vi "Connect.vi"(8 "error in (no error)":errorcluster) -> (0 "error out":errorcluster, 2 "controller":refnum<k24>)   [LabVIEW 2016]
uses:
  C:/Program Files (x86)/Aerotech/A3200/LabVIEW/2010/Bin/Aerotech.A3200.dll
  Program Files (x86)/Aerotech/A3200/LabVIEW/2010/Bin/Aerotech.A3200.dll
  C:/Program Files (x86)/Aerotech/A3200/LabVIEW/2010/Bin/Aerotech.A3200.LabVIEW.dll
  Program Files (x86)/Aerotech/A3200/LabVIEW/2010/Bin/Aerotech.A3200.LabVIEW.dll
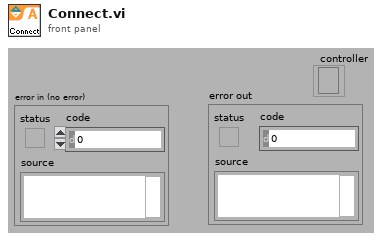
[diagram p1: front panel]
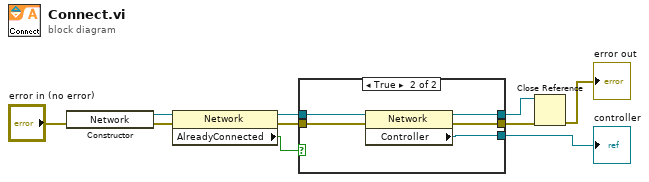
[diagram p0: block diagram]
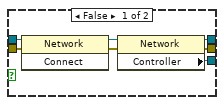
[diagram p2: hidden frame]
diagram:
  n1 = constructor class="Network"(error in="error in (no error)") -> (reference out=w8:refnum<k24>, error out=w7:errorcluster)  [unwired: 2 in, 1 out]
  n2 = property class="Network"(reference=w8, error in=w7) -> (reference out=w6:refnum<k24>, error out=w5:errorcluster, "AlreadyConnected"=w1:bool)
  n3 = case shown="True" w1 {
    tunnel: [w15 w19] -> w4
    tunnel: [w14 w20] -> w3
    tunnel: [w13 w18] -> w9
    tunnel: w6 -> [w12 w22]
    tunnel: w5 -> [w11 w21]
    frame False {
      n4 = invoke class="Network" method="Connect"(reference=w12, error in=w11) -> (reference out=w16:refnum<k24>, error out=w17:errorcluster)  [unwired: 1 in, 1 out]
      n5 = property class="Network"(reference=w16, error in=w17) -> (reference out=w14:refnum<k24>, error out=w15:errorcluster, "Controller"=w13:refnum<k24>)
    }
    frame True {
      n6 = property class="Network"(reference=w22, error in=w21) -> (reference out=w20:refnum<k24>, error out=w19:errorcluster, "Controller"=w18:refnum<k24>)
    }
  }
  "controller" <- w9
  n7 = Close Reference(reference=w3, error in (no error)=w4) -> (error out=→"error out":errorcluster)
